vi "Pololu.Mgr - Store Position.vi"(6 "Index":i32, 8 "error in (no error)":errorcluster, 9 "Pos(Deg)":dbl, 10 "Channel":u8, 11 "PololuCtrl in":refnum<class "PololuCtrl.lvclass">) -> (0 "error out":errorcluster, 2 "Device Config":T1[](array[typedef]), 3 "PololuCtrl out":refnum<class "PololuCtrl.lvclass">)   [LabVIEW 2018, in "PololuCtrl.lvclass"]
uses:
  PololuCtrl.lvclass
  SubVIs/Pololu.Device Config.ctl
  SubVIs/Pololu.Device Range Config.ctl
  PololuCtrl.lvclass/PololuCtrl.ctl
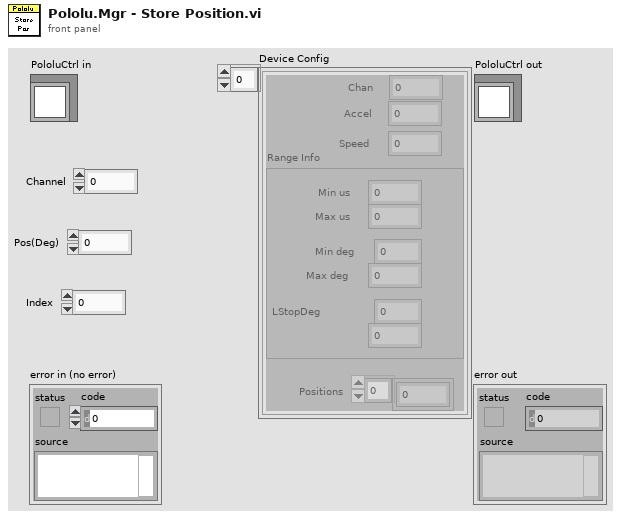
[diagram p1: front panel]
types:
  T1 = typedef "Pololu.Device Config.ctl" = cluster{"Chan":u8, "Accel":u16, "Speed":u16, "Positions":dbl[], "Range Info":T2}
  T2 = typedef "Pololu.Device Range Config.ctl" = cluster{"Min us":dbl, "Max us":dbl, "Min deg":dbl, "Max deg":dbl, "LStopDeg":dbl, "UStopDeg":dbl}
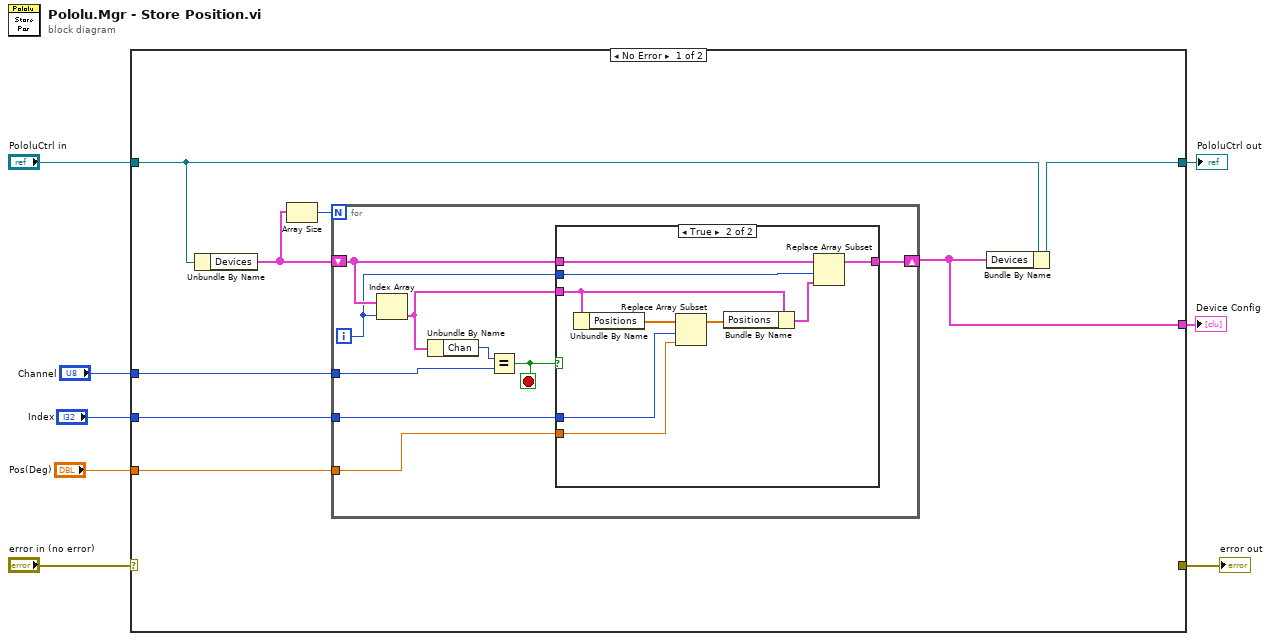
[diagram p0: block diagram]
diagram:
  n1 = case shown="No Error" "error in (no error)" {
    selector: "error in (no error)" -> [_ w37]
    tunnel: [_ w37] -> w7
    tunnel: [w14 w36] -> w5
    tunnel: "PololuCtrl in" -> [w15 w36]
    tunnel: "Channel" -> [w16 _]
    tunnel: "Pos(Deg)" -> [w11 _]
    tunnel: [w13 _] -> w2
    tunnel: "Index" -> [w12 _]
    frame No Error {
      n2 = Unbundle By Name(w15) -> ("Devices"=w10:T1[])
      n3 = Array Size(array=w10) -> (size(s)=w9:i32)
      n4 = for {
        N: w9 -> [_]
        shift-right: [w21] -> w13
        shift-left: w10 -> [w22]
        tunnel: w16 -> [w24]
        tunnel: w12 -> [w18]
        tunnel: w11 -> [w17]
        i -> [w20]
        stop <- w23 stop-if-true
        n5 = Index Array(array=w22, index=w20) -> (element=w19:T1)
        n6 = Unbundle By Name(w19) -> ("Chan"=w25:u8)
        n7 = Equal?(x=w25, y=w24) -> (x = y?=w23:bool)
        n8 = case shown="True" w23 {
          tunnel: w22 -> [w26 w35]
          tunnel: [w26 w34] -> w21
          tunnel: w20 -> [_ w33]
          tunnel: w19 -> [_ w32]
          tunnel: w18 -> [_ w29]
          tunnel: w17 -> [_ w28]
          frame False {
          }
          frame True {
            n9 = Unbundle By Name(w32) -> ("Positions"=w31:dbl[])
            n10 = Replace Array Subset(array=w31, new element=w28, index=w29) -> (w30:dbl[])
            n11 = Bundle By Name(cluster=w32, "Positions"=w30) -> (w27:T1)
            n12 = Replace Array Subset(array=w35, new element=w27, index=w33) -> (w34:T1[])
          }
        }
      }
      n13 = Bundle By Name(cluster=w15, "Devices"=w13) -> (w14:refnum<class "PololuCtrl.lvclass">)
    }
    frame Error {
    }
  }
  "error out" <- w7
  "PololuCtrl out" <- w5
  "Device Config" <- w2
